vi "Error Magic Sub.vi"(7 "QD Launch VI Panel?":bool, 8 "error in (no error)":errorcluster, 9 "Changed In":bool, 11 "VI in":refnum<vi>) -> (0 "error out":errorcluster, 1 "Changed Out":bool, 3 "VI out":refnum<vi>)   [LabVIEW 2017]
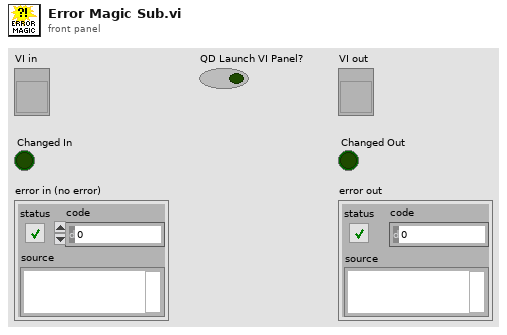
[diagram p1: front panel]
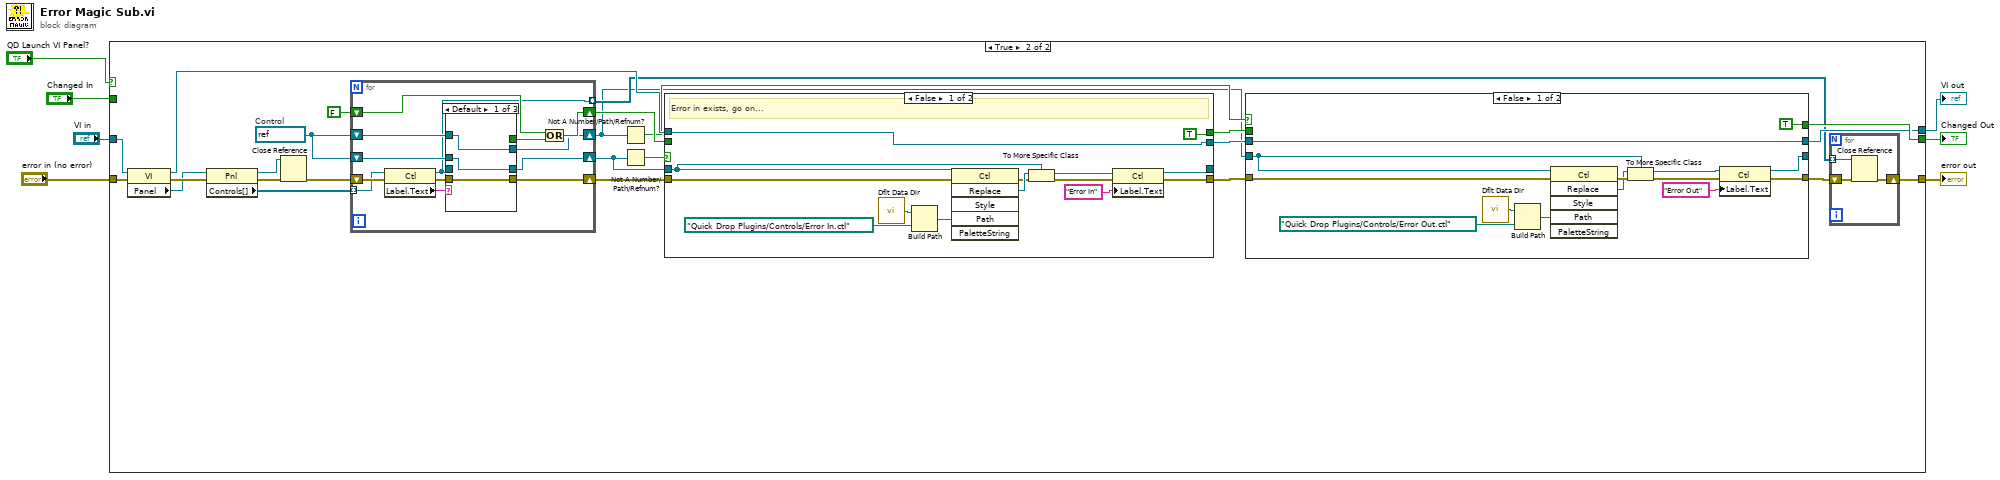
[diagram p0: block diagram]
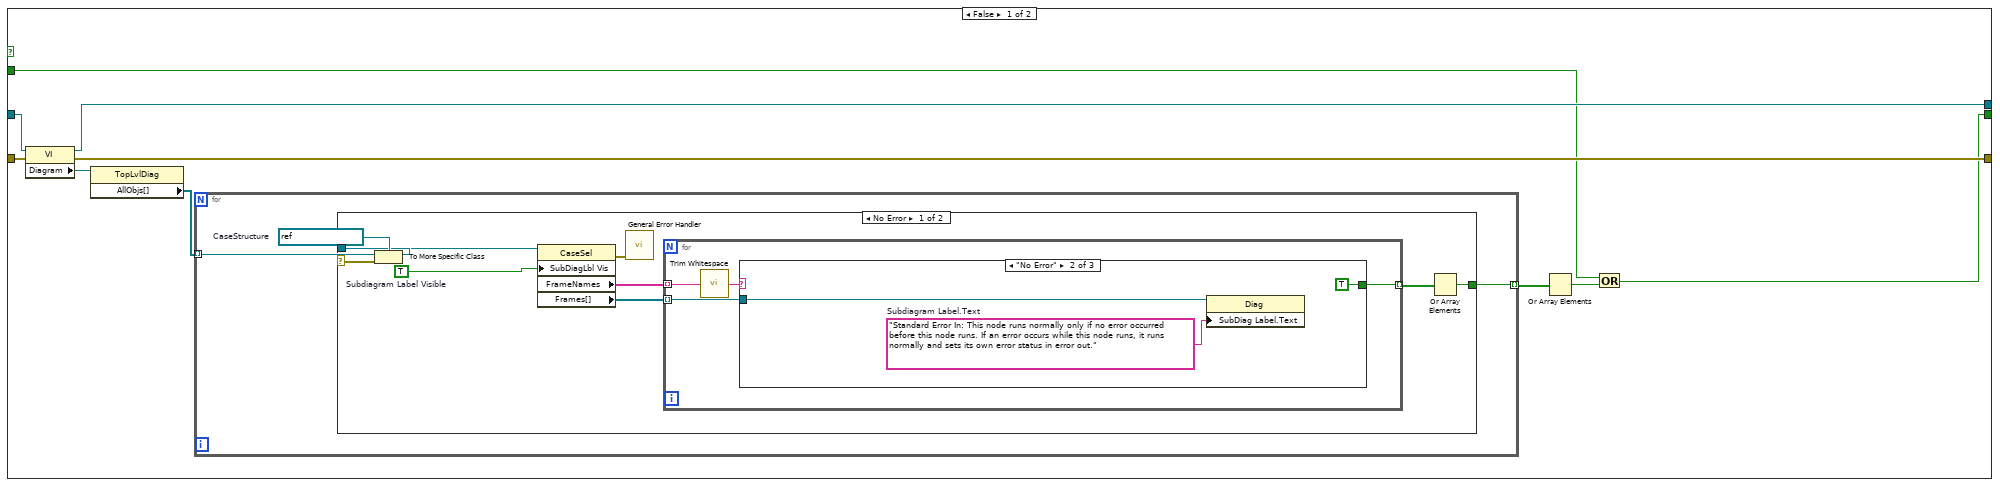
[diagram p2: hidden frame]
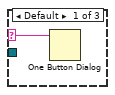
[diagram p3: hidden frame]
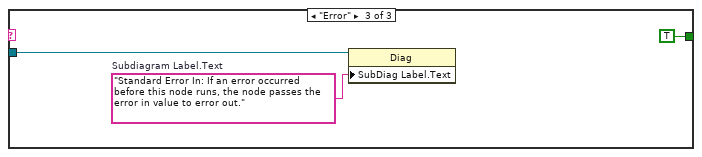
[diagram p4: hidden frame]
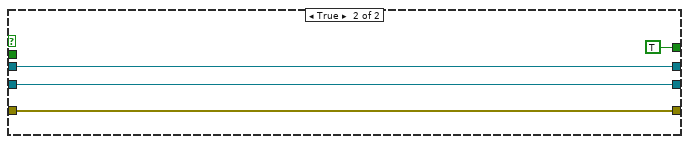
[diagram p6: hidden frame]
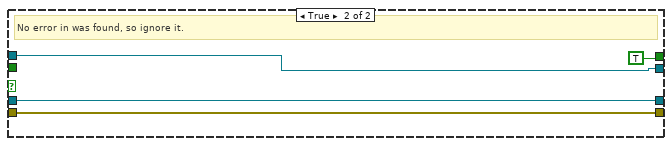
[diagram p7: hidden frame]
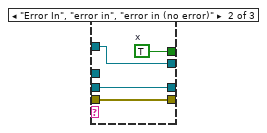
[diagram p8: hidden frame]
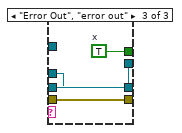
[diagram p9: hidden frame]
diagram:
  n1 = case shown="True" "QD Launch VI Panel?" {
    tunnel: "error in (no error)" -> [w17 w65]
    tunnel: [w16 w44] -> w4
    tunnel: "VI in" -> [w15 w63]
    tunnel: [w9 w52] -> w2
    tunnel: [w14 w48] -> w3
    tunnel: "Changed In" -> [w8 _]
    frame False {
      n2 = property class="VI"(reference=w15, error in=w17) -> (reference out=w14:refnum<vi>, error out=w16:errorcluster, "Diagram"=w13:refnum<vi>)
      n3 = property class="TopLvlDiag"(reference=w13) -> ("AllObjs[]"=w12:refnum<vi>[])  [unwired: 1 in, 2 out]
      n4 = for {
        tunnel: w12 -> [w19] mode=indexing
        tunnel: [w18] -> w11 mode=indexing
        w22 = refnum<vi> refnum  # CaseStructure
        n5 = To More Specific Class(target class=w22, reference=w19) -> (specific class reference=w21:refnum<vi>, error out=w20:errorcluster)  [unwired: 1 in]
        n6 = case shown="No Error" w20 {
          tunnel: w21 -> [w29 _]
          tunnel: [w23 _] -> w18
          frame No Error {
            w28 = TRUE  # Subdiagram Label Visible
            n7 = property class="CaseSel"(reference=w29, "SubDiagLbl Vis"=w28) -> (error out=w25:errorcluster, "FrameNames"=w27:string[], "Frames[]"=w26:refnum<vi>[])  [unwired: 1 in, 1 out]
            n8 = call <vilib>:"General Error Handler.vi"("error in (no error)"=w25) -> ()  [unwired: 10 in, 5 out]
            n9 = for {
              tunnel: w27 -> [w32] mode=indexing
              tunnel: w26 -> [w33] mode=indexing
              tunnel: [w31] -> w24 mode=indexing
              n10 = call <vilib>:"Trim Whitespace.vi"("string"=w32) -> ("trimmed string"=w30:string)  [unwired: 1 in]
              n11 = case shown="\"No Error\"" w30 {
                selector: w30 -> [w34 _ _]
                tunnel: w33 -> [_ w37 w40]
                tunnel: [_ TRUE TRUE] -> w31
                frame Default {
                  n12 = One Button Dialog(message=w34) -> ()  [unwired: 1 in, 1 out]
                }
                frame "No Error" {
                  w36 = "Standard Error In: This node runs normally only if no error occurred before this node runs. If an error occurs while this node runs, it runs normally and sets its own error status in error out."  # Subdiagram Label.Text
                  n13 = property class="Diag"(reference=w37, "SubDiag Label.Text"=w36) -> ()  [unwired: 1 in, 2 out]
                }
                frame "Error" {
                  w39 = "Standard Error In: If an error occurred before this node runs, the node passes the error in value to error out."  # Subdiagram Label.Text
                  n14 = property class="Diag"(reference=w40, "SubDiag Label.Text"=w39) -> ()  [unwired: 1 in, 2 out]
                }
              }
            }
            n15 = Or Array Elements(Boolean array=w24) -> (logical OR=w23:bool)
          }
          frame Error {
          }
        }
      }
      n16 = Or Array Elements(Boolean array=w11) -> (logical OR=w10:bool)
      n17 = Or(x=w8, y=w10) -> (x .or. y?=w9:bool)
    }
    frame True {
      w47 = refnum<vi> refnum  # Control
      n18 = property class="VI"(reference=w63, error in=w65) -> (reference out=w53:refnum<vi>, error out=w60:errorcluster, "Panel"=w59:refnum<vi>)
      n19 = property class="Pnl"(reference=w59, error in=w60) -> (reference out=w57:refnum<vi>, error out=w58:errorcluster, "Controls[]"=w62:refnum<vi>[])
      n20 = Close Reference(reference=w57, error in (no error)=w58) -> (error out=w64:errorcluster)
      n21 = for {
        shift-right: [w114] -> w54
        shift-left: w64 -> [w115]
        shift-right: [w116] -> w50
        shift-left: FALSE -> [w117]
        tunnel: w62 -> [w112] mode=indexing
        shift-right: [w109] -> w45
        shift-left: w47 -> [w108]
        shift-right: [w106] -> w41
        shift-left: w47 -> [w107]
        tunnel: [w105] -> w43 mode=indexing
        n22 = property class="Ctl"(reference=w112, error in=w115) -> (reference out=w105:refnum<vi>, error out=w111:errorcluster, "Label.Text"=w110:string)
        n23 = case shown="Default" w110 {
          tunnel: w105 -> [_ w124 w128]
          tunnel: w111 -> [w120 w123 w127]
          tunnel: [w120 w123 w127] -> w114
          tunnel: [_ w122 w126] -> w113
          tunnel: [w119 w124 w125] -> w109
          tunnel: w108 -> [w119 _ w125]
          tunnel: w107 -> [w118 w121 _]
          tunnel: [w118 w121 w128] -> w106
          frame Default {
          }
          frame "Error In", "error in", "error in (no error)" {
            w122 = TRUE  # x
          }
          frame "Error Out", "error out" {
            w126 = TRUE  # x
          }
        }
        n24 = Or(x=w117, y=w113) -> (x .or. y?=w116:bool)
      }
      n25 = Not A Number/Path/Refnum?(number/path/refnum=w41) -> (NaN/Path/Refnum?=w42:bool)
      n26 = Not A Number/Path/Refnum?(number/path/refnum=w45) -> (NaN/Path/Refnum?=w46:bool)
      n27 = case shown="False" w46 {
        tunnel: w54 -> [w99 w102]
        tunnel: w53 -> [w100 w104]
        tunnel: [w98 w102] -> w56
        tunnel: [w100 w104] -> w55
        tunnel: [TRUE TRUE] -> w51
        tunnel: w50 -> [_ _]
        tunnel: [w97 w101] -> _
        tunnel: w45 -> [w93 w101]
        frame False {
          # "Error in exists, go on..."
          n28 = call <vilib>:"Dflt Data Dir.vi"() -> ("App:Default Data Directory"=w89:path)
          n29 = Build Path(base path=w89, name or relative path=path "Quick Drop Plugins/Controls/Error In.ctl") -> (appended path=w87:path)
          n30 = invoke class="Ctl" method="Replace"(reference=w93, error in=w99, "Path"=w87) -> (error out=w92:errorcluster, "Replace"=w95:refnum<vi>)  [unwired: 3 in, 4 out]
          n31 = To More Specific Class(target class=w93, reference=w95, error in=w92) -> (specific class reference=w94:refnum<vi>, error out=w91:errorcluster)
          n32 = property class="Ctl"(reference=w94, error in=w91, "Label.Text"="Error In") -> (reference out=w97:refnum<vi>, error out=w98:errorcluster)
        }
        frame True {
          # "No error in was found, so ignore it."
        }
      }
      n33 = case shown="False" w42 {
        tunnel: w56 -> [w81 w84]
        tunnel: w55 -> [w82 w85]
        tunnel: [w80 w84] -> w49
        tunnel: [w82 w85] -> w48
        tunnel: [TRUE TRUE] -> w52
        tunnel: w51 -> [_ _]
        tunnel: [w79 w83] -> _
        tunnel: w41 -> [w75 w83]
        frame False {
          n34 = call <vilib>:"Dflt Data Dir.vi"() -> ("App:Default Data Directory"=w71:path)
          n35 = Build Path(base path=w71, name or relative path=path "Quick Drop Plugins/Controls/Error Out.ctl") -> (appended path=w69:path)
          n36 = invoke class="Ctl" method="Replace"(reference=w75, error in=w81, "Path"=w69) -> (error out=w77:errorcluster, "Replace"=w74:refnum<vi>)  [unwired: 3 in, 4 out]
          n37 = To More Specific Class(target class=w75, reference=w74, error in=w77) -> (specific class reference=w73:refnum<vi>, error out=w76:errorcluster)
          n38 = property class="Ctl"(reference=w73, error in=w76, "Label.Text"="Error Out") -> (reference out=w79:refnum<vi>, error out=w80:errorcluster)
        }
        frame True {
        }
      }
      n39 = for {
        tunnel: w43 -> [w66] mode=indexing
        shift-right: [w67] -> w44
        shift-left: w49 -> [w68]
        n40 = Close Reference(reference=w66, error in (no error)=w68) -> (error out=w67:errorcluster)
      }
    }
  }
  "error out" <- w4
  "VI out" <- w3
  "Changed Out" <- w2
